vi "Error message.vi"(8 "error in (no error)":errorcluster, 11 "Error description":string) -> (0 "error out":errorcluster)   [LabVIEW 2015]
panel:
  in  "OK Button":bool
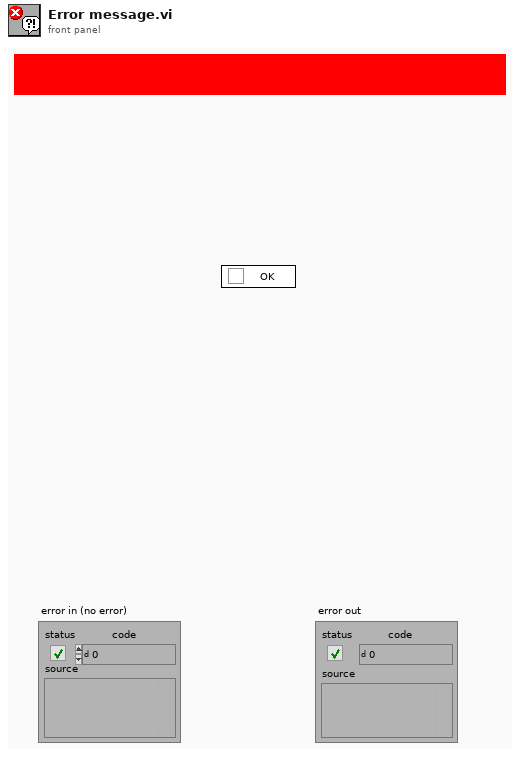
[diagram p1: front panel]
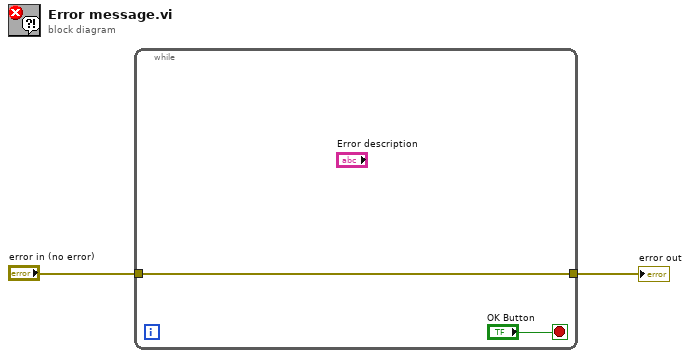
[diagram p0: block diagram]
diagram:
  n1 = while {
    tunnel: "error in (no error)" -> [w3]
    tunnel: [w3] -> w1
    stop <- "OK Button" stop-if-true
  }
  "error out" <- w1
